vi "isDone.vi"(8 "error in (no error)":errorcluster, 11 "IWaveform in":refnum<class "IWaveform.lvclass">) -> (0 "error out":errorcluster, 2 "isDone?":bool=TRUE, 3 "IWaveform out":refnum<class "IWaveform.lvclass">)   [LabVIEW 2015, in "IWaveform.lvclass"]
uses:
  IWaveform.lvclass
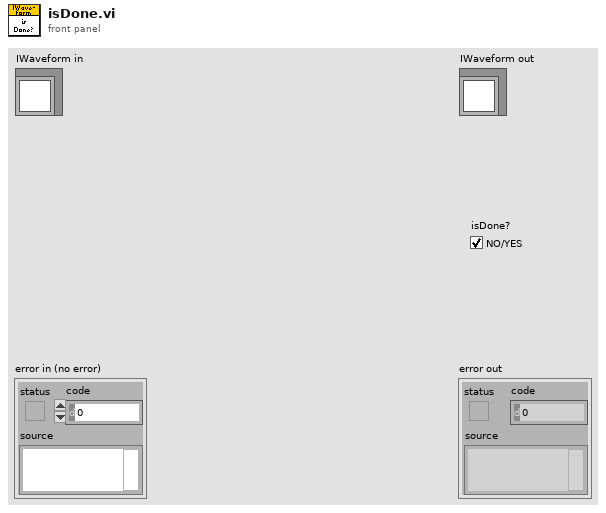
[diagram p1: front panel]
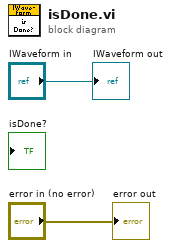
[diagram p0: block diagram]
diagram:
  "error out" <- "error in (no error)"
  "IWaveform out" <- "IWaveform in"
